vi "Write Command _Read Data_.vi"(8 "error in (no error)":errorcluster, 10 "Command \"Read Data\"":string, 11 "MultimeterControl in":refnum<class "MultimeterControl.lvclass">) -> (0 "error out":errorcluster, 3 "MultimeterControl out":refnum<class "MultimeterControl.lvclass">)   [LabVIEW 2018, in "MultimeterControl.lvclass"]
uses:
  MultimeterControl.lvclass
  MultimeterControl.lvclass/MultimeterControl.ctl
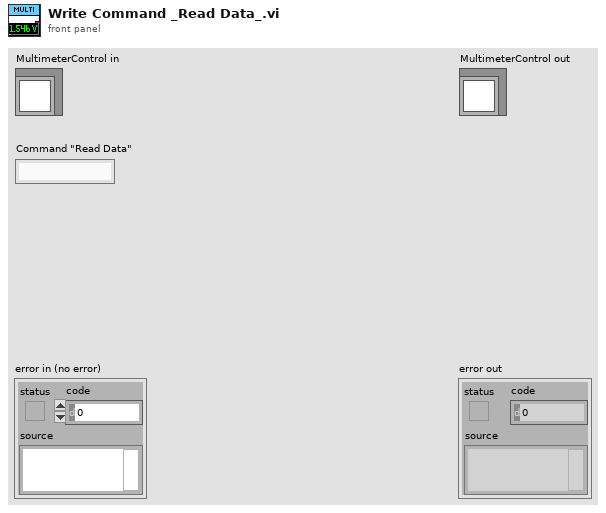
[diagram p1: front panel]
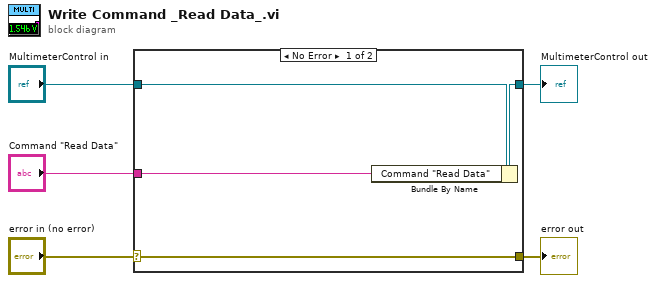
[diagram p0: block diagram]
diagram:
  n1 = case shown="No Error" "error in (no error)" {
    selector: "error in (no error)" -> [w9 w10]
    tunnel: [w9 w10] -> w4
    tunnel: [w7 w11] -> w2
    tunnel: "MultimeterControl in" -> [w8 w11]
    tunnel: "Command \"Read Data\"" -> [w6 _]
    frame No Error {
      n2 = Bundle By Name(cluster=w8, "Command \"Read Data\""=w6) -> (w7:refnum<class "MultimeterControl.lvclass">)
    }
    frame Error {
    }
  }
  "error out" <- w4
  "MultimeterControl out" <- w2
